vi "save_stored_position.vi"(8 "error in (no error)":errorcluster, 11 "StageDL090409Scaffold in":refnum<class "StageDL090409Scaffold.lvclass">) -> (0 "error out":errorcluster, 3 "StageDL090409Scaffold out":refnum<class "StageDL090409Scaffold.lvclass">)   [LabVIEW 2010, in "StageDL090409Scaffold.lvclass"]
uses:
  StageDL090409Scaffold.lvclass
  stored_data_cluster.ctl
  common/classes/SpaceVector/SpaceVector/SpaceVector.lvclass
  common/classes/Image/Image/Image.lvclass
  StageDL090409Scaffold.lvclass/StageDL090409Scaffold.ctl
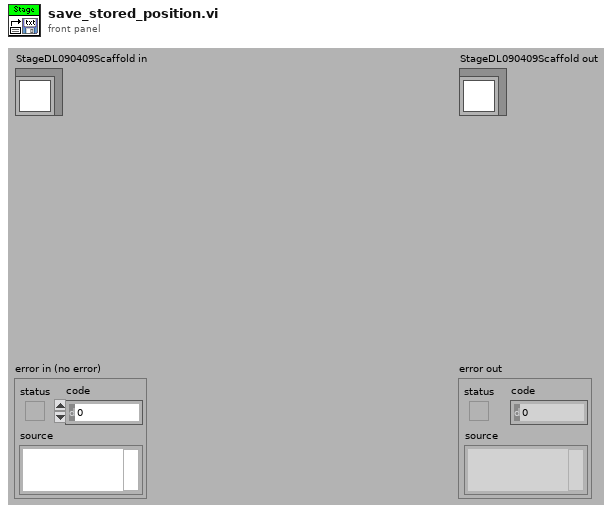
[diagram p1: front panel]
types:
  T1 = typedef "StageDL090409Scaffold.lvclass/stored_data_cluster.ctl" = cluster{"stored position":refnum<class "SpaceVector.lvclass">, "description":string, "position image":refnum<class "Image.lvclass">}
  T2 = cluster{"stored data array":T1[], "origin":refnum<class "SpaceVector.lvclass">}
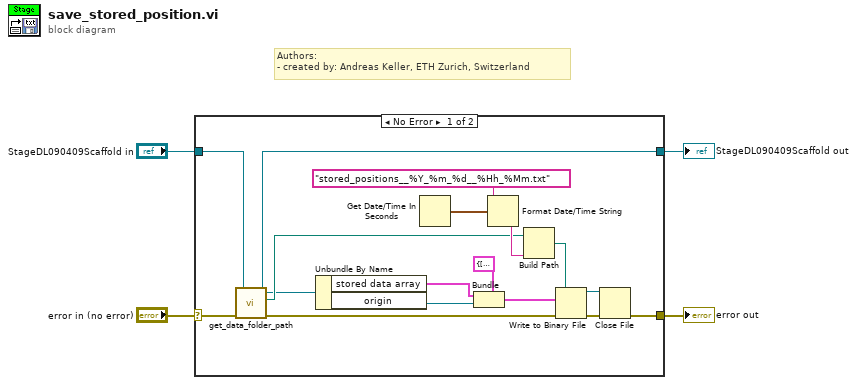
[diagram p0: block diagram]
diagram:
  # "Authors: \n- created by: Andreas Keller, ETH Zurich, Switzerland"
  n1 = case shown="No Error" "error in (no error)" {
    selector: "error in (no error)" -> [w15 w22]
    tunnel: [w10 w22] -> w3
    tunnel: [w8 w21] -> w1
    tunnel: "StageDL090409Scaffold in" -> [w14 w21]
    frame No Error {
      n2 = call-dynamic "get_data_folder_path.vi"("error in (no error)"=w15, "GenericComponent in"=w14) -> ("error out"=w16:errorcluster, "data folder path"=w13:path, "GenericComponent out"=w8:refnum<class "StageDL090409Scaffold.lvclass">)  [unwired: 7 in]
      n3 = Unbundle By Name(w8) -> ("stored data array"=w7:T1[], "origin"=w17:refnum<class "SpaceVector.lvclass">)
      n4 = Get Date/Time In Seconds() -> (seconds since 1Jan1904=w20:timestamp)
      n5 = Bundle(cluster=T2 {"stored data array"=[], "origin"=refnum} ("output cluster"), "stored data array"=w7, "origin"=w17) -> (w5:T2)
      n6 = Format Date/Time String(time format string (%c)="stored_positions__%Y_%m_%d__%Hh_%Mm.txt", seconds (now)=w20) -> (date/time string=w19:string)  [unwired: 1 in]
      n7 = Build Path(base path=w13, name or relative path=w19) -> (appended path=w12:path)
      n8 = Write to Binary File(file (use dialog)=w12, data=w5, error in=w16) -> (refnum out=w9:refnum<file>, error out=w11:errorcluster)  [unwired: 3 in, 1 out]
      n9 = Close File(refnum=w9, error in=w11) -> (error out=w10:errorcluster)  [unwired: 1 out]
    }
    frame Error {
    }
  }
  "error out" <- w3
  "StageDL090409Scaffold out" <- w1
